vi "Time-tv-ts-td.vi"(3 "计算参数 in":T1, 5 "SamplingRate":dbl) -> (0 "计算参数 out":T1)   [LabVIEW 2013]
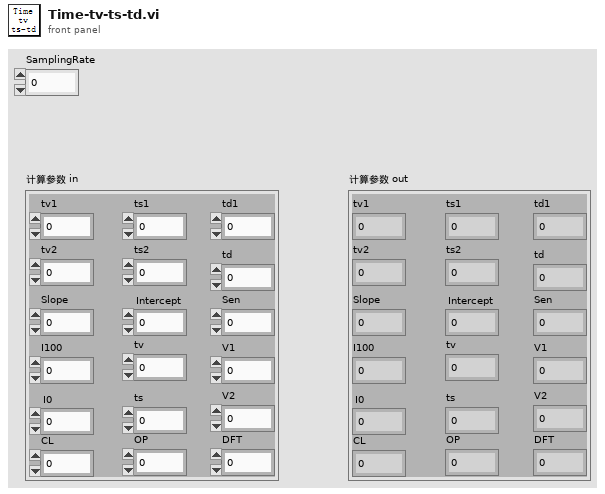
[diagram p1: front panel]
types:
  T1 = cluster{"tv1":dbl, "tv2":dbl, "tv":dbl, "ts1":dbl, "ts2":dbl, "ts":dbl, "td1":dbl, "td":dbl, "Slope":dbl, "Intercept":dbl, "I100":dbl, "I0":dbl, "Sen":dbl, "V1":dbl, "V2":dbl, "CL":dbl, "OP":dbl, "DFT":dbl}
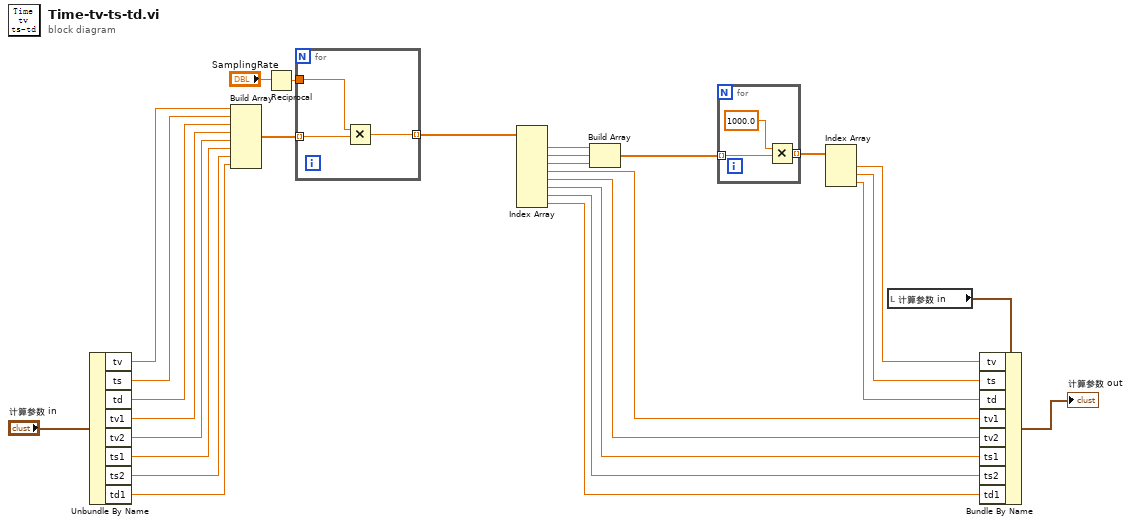
[diagram p0: block diagram]
diagram:
  n1 = Unbundle By Name("计算参数 in") -> ("tv"=w25:dbl, "ts"=w24:dbl, "td"=w23:dbl, "tv1"=w20:dbl, "tv2"=w19:dbl, "ts1"=w14:dbl, "ts2"=w13:dbl, "td1"=w12:dbl)
  n2 = Build Array(w25, w24, w23, w20, w19, w14, w13, w12) -> (w22:dbl[])
  n3 = Reciprocal(x="SamplingRate") -> (1/x=w16:dbl)
  n4 = for {
    tunnel: w22 -> [w31] mode=indexing
    tunnel: w16 -> [w30]
    tunnel: [w29] -> w21 mode=indexing
    n5 = Multiply(x=w30, y=w31) -> (x*y=w29:dbl)
  }
  n6 = Index Array(array=w21) -> (element #1=w8:dbl, element #2=w7:dbl, element #3=w6:dbl, element #4=w18:dbl, element #5=w17:dbl, element #6=w11:dbl, element #7=w10:dbl, element #8=w9:dbl)  [unwired: 8 in]
  n7 = Build Array(w8, w7, w6) -> (w5:dbl[])
  n8 = for {
    tunnel: w5 -> [w34] mode=indexing
    tunnel: [w33] -> w4 mode=indexing
    n9 = Multiply(x=1000.0, y=w34) -> (x*y=w33:dbl)
  }
  n10 = Index Array(array=w4) -> (element #1=w3:dbl, element #2=w2:dbl, element #3=w1:dbl)  [unwired: 3 in]
  n11 = local read "计算参数 in"() -> (w26:T1)
  n12 = Bundle By Name(cluster=w26, "tv"=w3, "ts"=w2, "td"=w1, "tv1"=w18, "tv2"=w17, "ts1"=w11, "ts2"=w10, "td1"=w9) -> (→"计算参数 out":T1)
